vi "启动测量模式选择对话框.vi"(9 "量程选择":enum16{"L", "H", "AUTO"}(ring), 10 "启动选择":u16(ring) items=["水样测试", "标样核查", "零点核查", "跨度核查", "空白测试", "加标回收", "平行样", "校零", "校标"], 11 "确定":bool) -> (2 "量程选择输出":enum16{"L", "H", "AUTO"}(ring), 3 "启动选择输出":u16(ring) items=["水样测试", "标样核查", "零点核查", "跨度核查", "空白测试", "加标回收", "平行样", "校零", "校标"])   [LabVIEW 2016, in "斯坦道CODMn.lvlib"]
uses:
  <vilib>/Utility/miscctls.llb/LVPointTypeDef.ctl
panel:
  in  "取消":bool
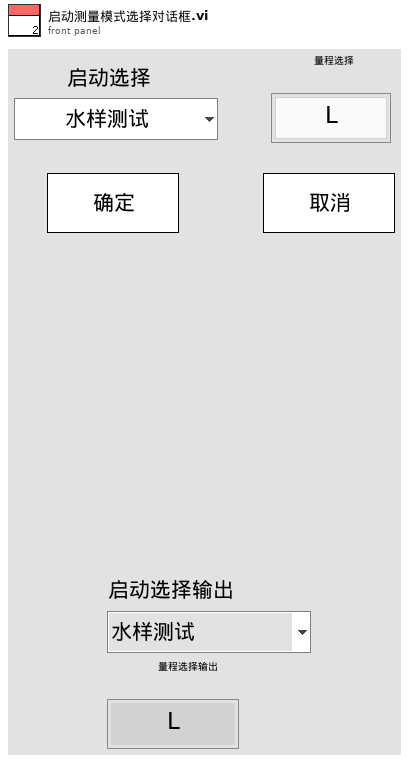
[diagram p1: front panel]
types:
  T1 = typedef "LVPointTypeDef.ctl" = cluster{"Horizontal":i16, "Vertical":i16}
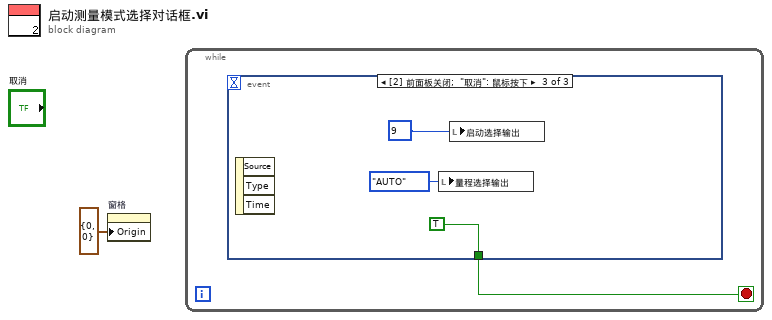
[diagram p0: block diagram]
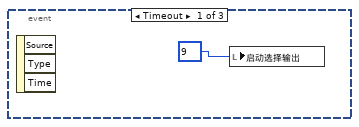
[diagram p2: hidden frame]
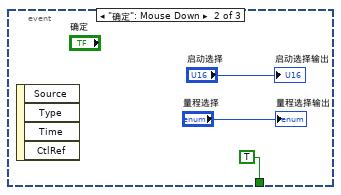
[diagram p3: hidden frame]
diagram:
  n1 = property on="窗格" class="Pane"("Origin"=T1 {"Horizontal"=0, "Vertical"=0} ("原点")) -> ()  [unwired: 2 in, 2 out]
  n2 = while {
    stop <- w2 stop-if-true
    n3 = event shown="[2] 前面板关闭;  \"取消\": 鼠标按下" {
      selector: _ -> [_ _ _]
      dyn-events: _ -> [_ _ _]
      timeout: _ -> [_ _ _]
      tunnel: [_ TRUE TRUE] -> w2
      event Timeout {
        w3 = u16 9 items=["水样测试", "标样核查", "零点核查", "跨度核查", "空白测试", "加标回收", "平行样", "校零", "校标", ""] ("启动选择 2")
        n4 = event-data() -> ()  [unwired: 1 in, 3 out]
        n5 = local write "启动选择输出"(w3) -> ()
      }
      event "确定": Mouse Down {
        n6 = event-data() -> ()  [unwired: 1 in, 4 out]
        "启动选择输出" <- "启动选择"
        "量程选择输出" <- "量程选择"
      }
      event Panel Close; "取消": Mouse Down {
        w8 = u16 9 items=["水样测试", "标样核查", "零点核查", "跨度核查", "空白测试", "加标回收", "平行样", "校零", "校标", ""] ("启动选择 2")
        n7 = event-data() -> ()  [unwired: 1 in, 3 out]
        n8 = local write "量程选择输出"(enum16{"L", "H", "AUTO"}."AUTO" ("量程选择输出")) -> ()
        n9 = local write "启动选择输出"(w8) -> ()
      }
    }
  }
